vi "Main Page.vi"(8 "error in (no error)":errorcluster, 11 "Node Ptr":T1 format="%.0x") -> (0 "error out":errorcluster)   [LabVIEW 2019, in "Reset Hardware System Explorer.lvlib"]
uses:
  Reset Hardware System Explorer.lvlib
  <vilib>/NI VeriStand/Custom Device API/Custom Device Item Ref.ctl
  Shared/Constants.vi
  <vilib>/NI/NI VeriStand Advanced SysDef API/_SubVIs/SysDef.Property.Get.Boolean.vi
  <vilib>/NI/NI VeriStand Advanced SysDef API/_SubVIs/SysDef.Property.Set.Boolean.vi
  <vilib>/NI VeriStand/Custom Device API/Custom Device API.lvlib
  <vilib>/NI/NI VeriStand Advanced SysDef API/SysDef API/Advanced System Definition.lvlib
  Shared/Reset Hardware Shared.lvlib
panel:
  in  "Reset XNET":bool=TRUE
  in  "Reset AO":bool=TRUE
  out "Version":string
  in  "SHDocVw.IWebBrowser":refnum<k7>(container)
  in  "Specific Header":cluster{"Section Name":string}={"Section Name"="Custom Device Item Settings"}
  in  "General Header":cluster{"Section Name":string}={"Section Name"="General Custom Device Settings"}
  in  "Description":string
  in  "Name":string
  # "On E Series, S Series, and AO Series devices, NI-DAQmx Reset does not alter the AO channels. They continue to generate the DC voltage you last set them to. Enable this property to reset all AO channels to 0 Volts."
  # "Self-Testing resets the firmware of the device occasionally. Enable this property to reset all NI-XNET devices by performing a self-test."
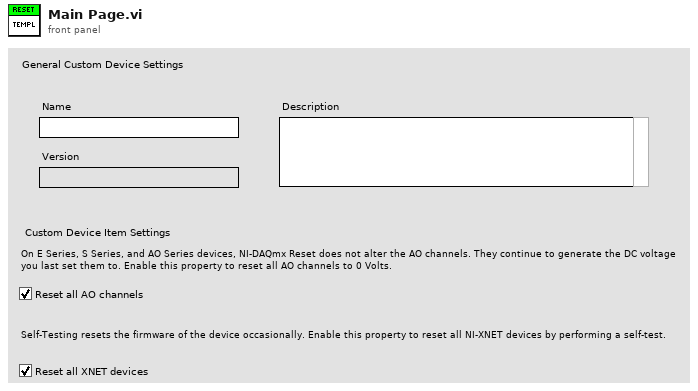
[diagram p1: front panel]
types:
  T1 = typedef "Custom Device API.lvlib/Custom Device Item Ref.ctl" = u64
  T2 = typedef "Custom Device API.lvlib/Custom Device Item Info.ctl" = cluster{"Name":string, "Is Channel":bool, "GUID":string, "Is Waveform":bool}
  T3 = typedef "Custom Device API.lvlib/Custom Device Commands.ctl" = enum16{"Default", "Item renamed", "Shutdown", "Dynamic button pressed"}
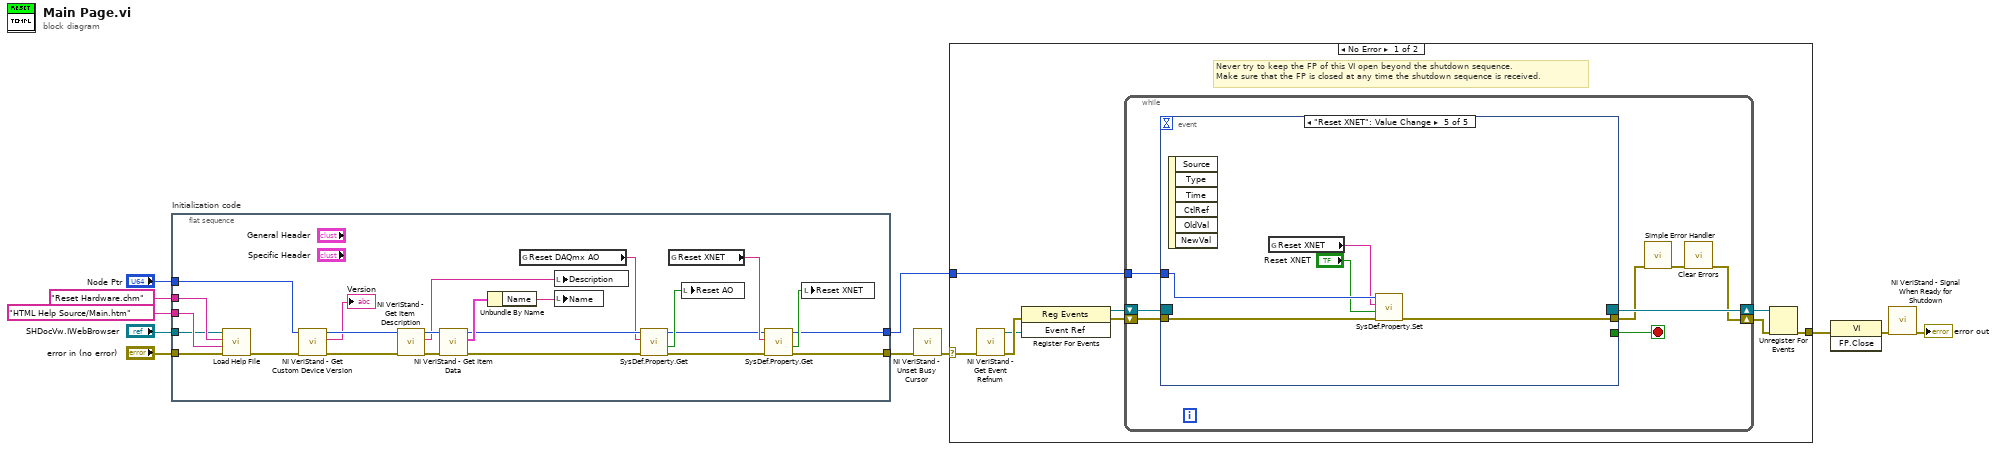
[diagram p0: block diagram]
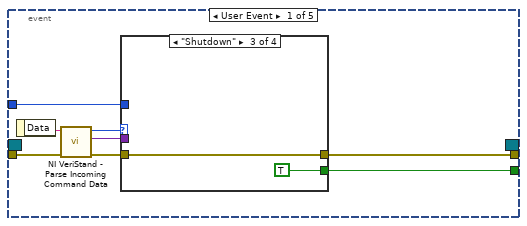
[diagram p2: hidden frame]
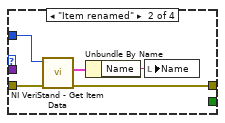
[diagram p4: hidden frame]
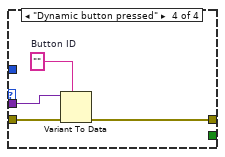
[diagram p5: hidden frame]
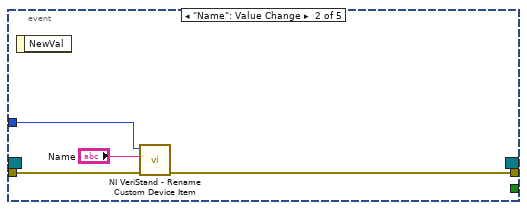
[diagram p6: hidden frame]
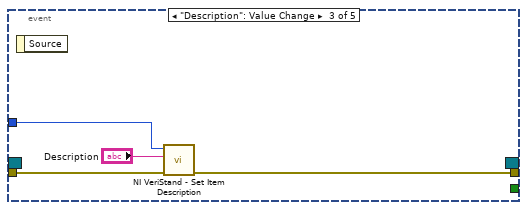
[diagram p7: hidden frame]
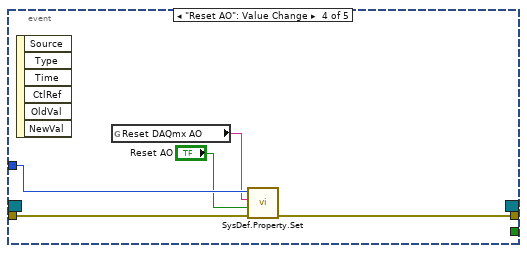
[diagram p8: hidden frame]
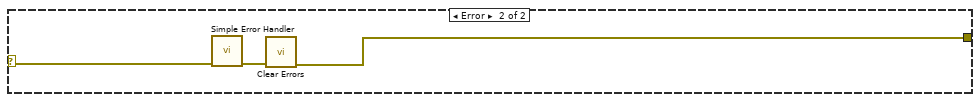
[diagram p9: hidden frame]
diagram:
  n1 = flat-sequence "Initialization code" {
    tunnel: "error in (no error)" -> [w26]
    tunnel: "Node Ptr" -> [w32]
    tunnel: [w12] -> w7
    tunnel: [w13] -> w4
    tunnel: "SHDocVw.IWebBrowser" -> [w22]
    tunnel: "HTML Help Source/Main.htm" ("HTML File") -> [w23]
    tunnel: "Reset Hardware.chm" ("CD_CHM_FileName") -> [w24]
    frame #0 {
      n2 = call "Load Help File.vi"("error in (no error)"=w26, "HTML File to Load"=w23, "Main CHM File"=w24, "Browser"=w22) -> ("error out"=w25:errorcluster)  [unwired: 7 in]
      n3 = call <vilib>:"NI VeriStand - Get Custom Device Version.vi"("error in (no error)"=w25, "Device Ref in"=w32) -> ("error out"=w31:errorcluster, "Value"=→"Version":string, "Device Ref out"=w30:T1)  [unwired: 7 in]
      n4 = call <vilib>:"NI VeriStand - Get Item Description.vi"("error in (no error)"=w31, "Item Ref in"=w30) -> ("error out"=w34:errorcluster, "Description"=w27:string, "Item Ref out"=w35:T1)  [unwired: 7 out]
      n5 = call <vilib>:"NI VeriStand - Get Item Data.vi"("error in (no error)"=w34, "Item Ref in"=w35) -> ("error out"=w20:errorcluster, "Item Info"=w33:T2, "Item Ref out"=w21:T1)  [unwired: 7 out]
      n6 = Unbundle By Name(w33) -> ("Name"=w28:string)
      n7 = global read "Constants.vi" "Reset DAQmx AO"() -> (w19:string)
      n8 = local write "Description"(w27) -> ()
      n9 = local write "Name"(w28) -> ()
      n10 = call-poly <vilib>:"SysDef.Property.Get.vi"("error in (no error)"=w20, "Property Name"=w19, "nodeID"=w21) -> ("error out"=w14:errorcluster, "Value out"=w18:bool, "nodeID out"=w15:u64)  [unwired: 5 in, 1 out]
      n11 = global read "Constants.vi" "Reset XNET"() -> (w16:string)
      n12 = local write "Reset AO"(w18) -> ()
      n13 = call-poly <vilib>:"SysDef.Property.Get.vi"("error in (no error)"=w14, "Property Name"=w16, "nodeID"=w15) -> ("error out"=w12:errorcluster, "Value out"=w17:bool, "nodeID out"=w13:u64)  [unwired: 5 in, 1 out]
      n14 = local write "Reset XNET"(w17) -> ()
    }
  }
  n15 = call <vilib>:"NI VeriStand - Unset Busy Cursor.vi"("error in (no error)"=w7) -> ("error out"=w6:errorcluster)  [unwired: 10 out]
  n16 = case shown="No Error" w6 {
    selector: w6 -> [w36 w93]
    tunnel: [w41 w91] -> w11
    tunnel: w4 -> [w37 _]
    frame No Error {
      # "Never try to keep the FP of this VI open beyond the shutdown sequence.\nMake sure that the FP is closed at any time the shutdown sequence is received."
      n17 = call <vilib>:"NI VeriStand - Get Event Refnum.vi"("error in (no error)"=w36) -> ("error out"=w44:errorcluster, "Event Ref"=w40:refnum<user-event>)  [unwired: 9 out]
      n18 = register-events(error in=w44, w40) -> (reference out=w38:refnum<event-registration>, error out=w39:errorcluster)  [unwired: 1 in]
      n19 = while {
        tunnel: w37 -> [w48]
        shift-right: [w45] -> w42
        shift-left: w39 -> [w51]
        shift-right: [w52] -> w43
        shift-left: w38 -> [w50]
        stop <- w49 stop-if-true
        n20 = event shown="[4] \"Reset XNET\": Value Change" {
          selector: w50 -> [_ _ _ _ _]
          dyn-events: [_ _ _ _ _] -> w52
          timeout: _ -> [_ _ _ _ _]
          tunnel: w51 -> [w60 w76 w79 w85 w90]
          tunnel: [w56 _ _ _ _] -> w49
          tunnel: [w55 w75 w78 w84 w89] -> w47
          tunnel: w48 -> [w54 w74 w80 w83 w88]
          event User Event {
            n21 = event-data() -> ("Data"=w59:string)  [unwired: 1 out]
            n22 = call <vilib>:"NI VeriStand - Parse Incoming Command Data.vi"("error in (no error)"=w60, "Incoming data"=w59) -> ("error out"=w58:errorcluster, "Outgoing data"=w53:variant, "Action"=w57:T3)  [unwired: 7 out]
            n23 = case shown="\"Shutdown\"" w57 {
              tunnel: w58 -> [w61 w66 w67 w72]
              tunnel: [_ _ TRUE _] -> w56
              tunnel: [w61 w63 w67 w69] -> w55
              tunnel: w54 -> [_ w65 _ _]
              tunnel: w53 -> [_ _ _ w71]
              frame "Default", Default {
              }
              frame "Item renamed" {
                n24 = call <vilib>:"NI VeriStand - Get Item Data.vi"("error in (no error)"=w66, "Item Ref in"=w65) -> ("error out"=w63:errorcluster, "Item Info"=w64:T2)  [unwired: 8 out]
                n25 = Unbundle By Name(w64) -> ("Name"=w62:string)
                n26 = local write "Name"(w62) -> ()
              }
              frame "Shutdown" {
              }
              frame "Dynamic button pressed" {
                w70 = ""  # Button ID
                n27 = Variant To Data(error in=w72, type=w70, Variant=w71) -> (error out=w69:errorcluster)  [unwired: 1 out]
              }
            }
          }
          event "Name": Value Change {
            n28 = event-data() -> ()  [unwired: 2 out]
            n29 = call <vilib>:"NI VeriStand - Rename Custom Device Item.vi"("error in (no error)"=w76, "New Name"="Name", "Item Ref in"=w74) -> ("error out"=w75:errorcluster)  [unwired: 1 in, 7 out]
          }
          event "Description": Value Change {
            n30 = event-data() -> ()  [unwired: 2 out]
            n31 = call <vilib>:"NI VeriStand - Set Item Description.vi"("error in (no error)"=w79, "Description"="Description", "Item Ref in"=w80) -> ("error out"=w78:errorcluster)  [unwired: 8 out]
          }
          event "Reset AO": Value Change {
            n32 = event-data() -> ()  [unwired: 7 out]
            n33 = global read "Constants.vi" "Reset DAQmx AO"() -> (w82:string)
            n34 = call-poly <vilib>:"SysDef.Property.Set.vi"("error in (no error)"=w85, "Value"="Reset AO", "Property Name"=w82, "nodeID"=w83) -> ("error out"=w84:errorcluster)  [unwired: 6 in, 1 out]
          }
          event "Reset XNET": Value Change {
            n35 = event-data() -> ()  [unwired: 7 out]
            n36 = global read "Constants.vi" "Reset XNET"() -> (w87:string)
            n37 = call-poly <vilib>:"SysDef.Property.Set.vi"("error in (no error)"=w90, "Value"="Reset XNET", "Property Name"=w87, "nodeID"=w88) -> ("error out"=w89:errorcluster)  [unwired: 6 in, 1 out]
          }
        }
        n38 = call <vilib>:"Simple Error Handler.vi"("error in (no error)"=w47) -> ("error out"=w46:errorcluster)  [unwired: 1 in, 7 out]
        n39 = call <vilib>:"Clear Errors.vi"("error in (no error)"=w46) -> ("error out"=w45:errorcluster)  [unwired: 1 in, 5 out]
      }
      n40 = Unregister For Events(event registration refnum=w43, error in=w42) -> (error out=w41:errorcluster)
    }
    frame Error {
      n41 = call <vilib>:"Simple Error Handler.vi"("error in (no error)"=w93) -> ("error out"=w92:errorcluster)  [unwired: 1 in, 7 out]
      n42 = call <vilib>:"Clear Errors.vi"("error in (no error)"=w92) -> ("error out"=w91:errorcluster)  [unwired: 1 in, 5 out]
    }
  }
  n43 = invoke class="VI" method="FP.Close"(error in=w11) -> (error out=w10:errorcluster)  [unwired: 2 in, 2 out]
  n44 = call <vilib>:"NI VeriStand - Signal When Ready for Shutdown.vi"("error in (no error)"=w10) -> ("error out"=→"error out":errorcluster)  [unwired: 10 out]
